vi "FrontPanel.vi"() -> ()   [LabVIEW 2013]
doc: "This VI controls the blindpanel type GHS-2T-1T-700 for a CryoFree DR. Automatization control is embedded in the blindpanel. Keys can be manipulated from within this VI."
uses:
  Lib/Lib.llb/ErrCodeStatusLkup.vi
  Lib/Lib.llb/Pfeiffer Vacuum.lvlib
panel:
  out "millisecond timer value":u32
  out "Timer 2":u32
  out "Timer 1":u32
  out "Cur Path":path
  in  "Start":bool caption="stop"
  in  "stop":bool
  in  "Side Panel":enum32{"Main", "HW Settings"}(tab)=enum."HW Settings"
  out "Sensors Status":T1={"String 8"="OK", "String 9"="OK", "String 10"="OK", "String 11"="OK", "String 12"="OK", "String 13"="OK"}
  out "cluster":T2 {"Channel 1" format="%-7.2e mbar"; "Channel 1" format="%-7.2e mbar"; "Channel 1" format="%-7.2e mbar"; "Channel 1" format="%-7.2e mbar"; "Channel 1" format="%-7.2e mbar"; "Channel 1" format="%-7.2e mbar"}
  out "Cluster":T3={"String 2"="\"\"", "String 3"="", "String 4"="", "String 5"="", "String 6"="", "String 7"=""}
  in  "S1":enum32{"Page 1"}(tab)
  out "Error code":string
  in  "Reset Error":bool
  out "Turbo T":T4
  out "Turbo IW":cluster{"I:":string, "P:":string}
  out "Turbo status":T5={"uA"="000", "Set Speed"=FALSE, "On"=FALSE, "Error"=FALSE}
  in  "S2":enum32{"Page 1"}(tab)
  out "Error code":string
  in  "Reset Error 2":bool
  out "Turbo T 2":T4
  out "Turbo IW 2":cluster{"I:":string, "P:":string}
  out "Turbo status 2":T5={"uA"="000", "Set Speed"=FALSE, "On"=FALSE, "Error"=FALSE}
  in  "Data Logging \nOptions":T6={"Plot data "=TRUE, "Every"=1.0, "Save to log"=TRUE, "Every  2"=1.0, "AVS_Path 2"=path "C:/avs-47", "AVS_FName"="logFP", "Filename suffix"="_%Y-%m-%d-%H-%M-%S", "NewFevery"=7, "Time Units"=enum."Days", "Date Format"="%Y-%m-%d %H:%M:%S", "Averages"=4} {"Every  2" format="%#_g min"; "Every" format="%#_g min"}
  in  "P6&7 Settings":T7={"P6 low"=20, "P6 high"=1600, "P7 low"=20, "P7 high"=1610, "Delay preset"=86400.0} {"Delay preset" format="%#_g minutes"}
  in  "P5 Settings":cluster{"P6 low":u16, "P6 high":u16}={"P6 low"=20, "P6 high"=1000}
  in  "NCP5 Settings":T8={"P6 low"=20, "P6 high"=1000, "P7 low"=20}
  out "P6&7 limits":T9={"P6 low"=20, "P6 high"=20, "P7 low"=20, "P7 high"=20}
  out "P5 limits":cluster{"P5 low":u16, "P5 high":u16}={"P5 low"=20, "P5 high"=20}
  out "NCP5 limits":T10={"P5 low"=20, "P5 med"=20, "P5 high"=20}
  in  "SET VALUES":bool
  in  "ADC Scaling":T11={"Front panel ADC scaling factors"={"P1"=2500.0, "P2"=2500.0, "P3"=2500.0, "P4"=2500.0, "P5"=2500.0, "P6"=2500.0, "P7"=2500.0, "Flow meter"=256.0, "PC"=10000.0}} {"Front panel ADC scaling factors"."Flow meter" format="%#.4f"}
  in  "Configuration":T12={"FP port"="COM7", "MG port"="COM9", "PT Enabled?"=FALSE, "MG  channel P8"=65535, "Stop auto recovery if still is empty"=FALSE, "PT port"="COM2", "MG Enabled?"=FALSE, "Type"=enum."Wet", "Slave Address"=16, "S1 Enabled?"=FALSE, "S1 port"="COM2", "S2 Enabled?"=FALSE, "S2 port"="COM2", "Device address S1"=1, "Device address S2"=2} {"MG  channel P8" items=["Channel 1", "Channel 2", "Channel 3", "Channel 4", "Channel 5", "Channel 6"]; "Slave Address" min=16 max=126 step=1}
  in  "Error Panel":enum32{"Page 1", "Page 2"}(tab)
  out "PT error":errorcluster
  out "FP error":errorcluster
  out "Sensor ERROR":string="No error"
  out "MaxiGauge ERROR":string="No error"
  out "MG error":errorcluster
  in  "Autoconf":bool caption="Autoconfigure"
  out "MG Data":dbl[](array[numeric]) format="%.3e"
  out "FP Data":sgl[](array[numeric]) format="%.2f"
  out "FP Status bits":u32[](array[numeric])
  out "Maxigauge ID":string
  out "PT Data":dbl[](array[numeric])
  in  "Pressures Panel":enum32{"Page 1", "Page 2"}(tab)
  out "PC":sgl format="%.1f"
  out "P1":sgl format="%.1f"
  out "P2":sgl format="%.1f"
  out "P3":sgl format="%.1f"
  out "P4":sgl format="%.1f"
  out "P5":sgl format="%.1f"
  out "P6":sgl format="%.1f"
  out "P7":sgl format="%.1f"
  out "Flow":sgl format="%#_4f"
  out "P5 Alarm":bool
  out "Pstill (P8)":dbl format="%.3f"
  out "Attempts Counter":u16
  in  "Main Panel":T13(tab)
  out "String":string
  out "String 3":string
  out "Mode":u16(ring) items=["AUTO MODE OFF", "START", "CONDENSING 3He", "CONDENSING 4He", "NORMAL CIRCULATION", "RECOVERY OF THE MIXTURE", "RECOVERY: BLOCKAGE OR OVERPRESSURE"]
  out "FLOW":sgl format="%#_3f"
  out "P5":sgl
  out "P4":sgl
  out "P3":sgl
  out "P1":sgl
  out "P2":sgl
  out "3He":sgl(slide) min=0 max=2 scale=0.0..2000.0 scale format="%.2f"
  out "4He":sgl(slide) min=0 max=2 scale=0.0..2000.0 scale format="%.2f"
  out "Panel ID":string
  out "Revision":string caption="V"
  in  "Tab Control 4":enum32{"OLD", "NEW"}(tab)
  in  "Buttons":T14
  out "LEDs":T15
  out "PC":sgl caption="P COMP"
  in  "Buttons 2":T14
  out "LEDs 2":T16
  in  "PT Plots Select":T17
  out "PT Error Code":i32
  out "PT Status":string="NO ERROR"
  in  "Time delay":u16=60 format="%.0f s"
  in  "Attempts":u16=6
  in  "Restart PT on Error?":bool
  in  "Reset MIN/MAX":bool
  out "Motor Current":i32(slide) scale=0.0..50.0 scale format="%#.0f"
  out "He Pressure":cluster{dbl, dbl, dbl, dbl, dbl, dbl}(knob) scale=0.0..400.0
  out "Oil Temp":cluster{dbl, dbl, dbl, dbl}(slide)={0.0, 0.0, 0.0, 48.8} scale=0.0..55.0
  out "He Temp":cluster{dbl, dbl, dbl, dbl}(slide)={0.0, 0.0, 0.0, 87.8} scale=0.0..95.0
  out "Out Water Temp":cluster{dbl, dbl, dbl, dbl}(slide)={0.0, 0.0, 0.0, 52.0} scale=0.0..60.0
  in  "PT start":bool
  in  "PT stop":bool
  out "In Water Temp":cluster{dbl, dbl, dbl, dbl}(slide)={0.0, 0.0, 0.0, 29.4} scale=0.0..35.0
  out "PT Control":u16(ring) items=["Compressor OFF", "Compressor ON", ""]
  out "Error Log":string[][](table)
  out "PT Status":cluster{"Time":dbl[], "Value":dbl[]}[](graph)
  in  "MG Plots Select":T17
  in  "FP Plots Select":T17
  out "MaxiGauge":cluster{"Time":dbl[], "Value":dbl[]}[](graph)
  out "Front Panel":cluster{"Time":dbl[], "Value":dbl[]}[](graph)
  # "MaxiGauge"
  # "#"
  # "Name"
  # "Pressure"
  # "Status"
  # "1"
  # "2"
  # "3"
  # "4"
  # "5"
  # "6"
  # "Turbo1 (S1)"
  # "°C"
  # "°C"
  # "°C"
  # "°C"
  # "°C"
  # "A"
  # "W"
  # "Hz"
  # "Turbo2 (S2)"
  # "°C"
  # "°C"
  # "°C"
  # "°C"
  # "°C"
  # "A"
  # "W"
  # "Hz"
  # "Data Logging and Plotting"
  # "Automatic mode pressure limits"
  # "Warning: these values influence the automatic \nmode operation of the GHS. Please consult with Leiden Cryogenics before changing them."
  # "Front panel ADC scaling factors"
  # "NAME"
  # "EPROM"
  # "NEW"
  # "DESCRIPTION"
  # "Stop condensing 4He"
  # "Stop recovering 4He"
  # "Stop condensing 3He"
  # "Stop recovering 3He"
  # "Condensing->open 12"
  # "Condensing->close 9/12"
  # "NC->open second line"
  # "NC->start MC"
  # "NC->open aux. trap"
  # "MaxiGauge"
  # "Pulse Tube"
  # "Turbo 1 (S1) (Pfeiffer HiPACE only)"
  # "Turbo2 (S2) (Pfeiffer HiPACE only)"
  # "Front Panel"
  # "Front Panel Status"
  # "MaxiGauge Status"
  # "Pulse Tube Status"
  # "Leiden Cryogenics"
  # "to 3He\nin-1"
  # "to 3He\nin-2"
  # "from still"
  # "to \nair"
  # "N.C."
  # "from\novc"
  # "from\nivc"
  # "P8"
  # "AUX 1"
  # "MIXTURE\nCOMPRESSOR"
  # "M2"
  # "P6"
  # "M3"
  # "M1"
  # "AUX PORT-1"
  # "P7"
  # "TRAP"
  # "AUX TRAP"
  # "to 3He\nin-1"
  # "to 3He\nin-2"
  # "from still"
  # "To \nAir"
  # "From\nIVC"
  # "to 3He\nin-1"
  # "to 3He\nin-2"
  # "from still"
  # "to \nair"
  # "N.C."
  # "from\novc"
  # "from\nivc"
  # "Leiden Cryogenics"
  # "to 3He\nin-1"
  # "to 3He\nin-2"
  # "from still"
  # "to \nair"
  # "N.C."
  # "from\novc"
  # "from\nivc"
  # "P8"
  # "P8"
  # "M2"
  # "P6"
  # "M3"
  # "TRAP"
  # "AUX TRAP"
  # "M1"
  # "AUX PORT-1"
  # "P7"
  # "to 3He\nin-1"
  # "to 3He\nin-2"
  # "from still"
  # "To \nAir"
  # "From\nIVC"
  # "to 3He\nin-1"
  # "to 3He\nin-2"
  # "from still"
  # "to \nair"
  # "N.C."
  # "from\novc"
  # "from\nivc"
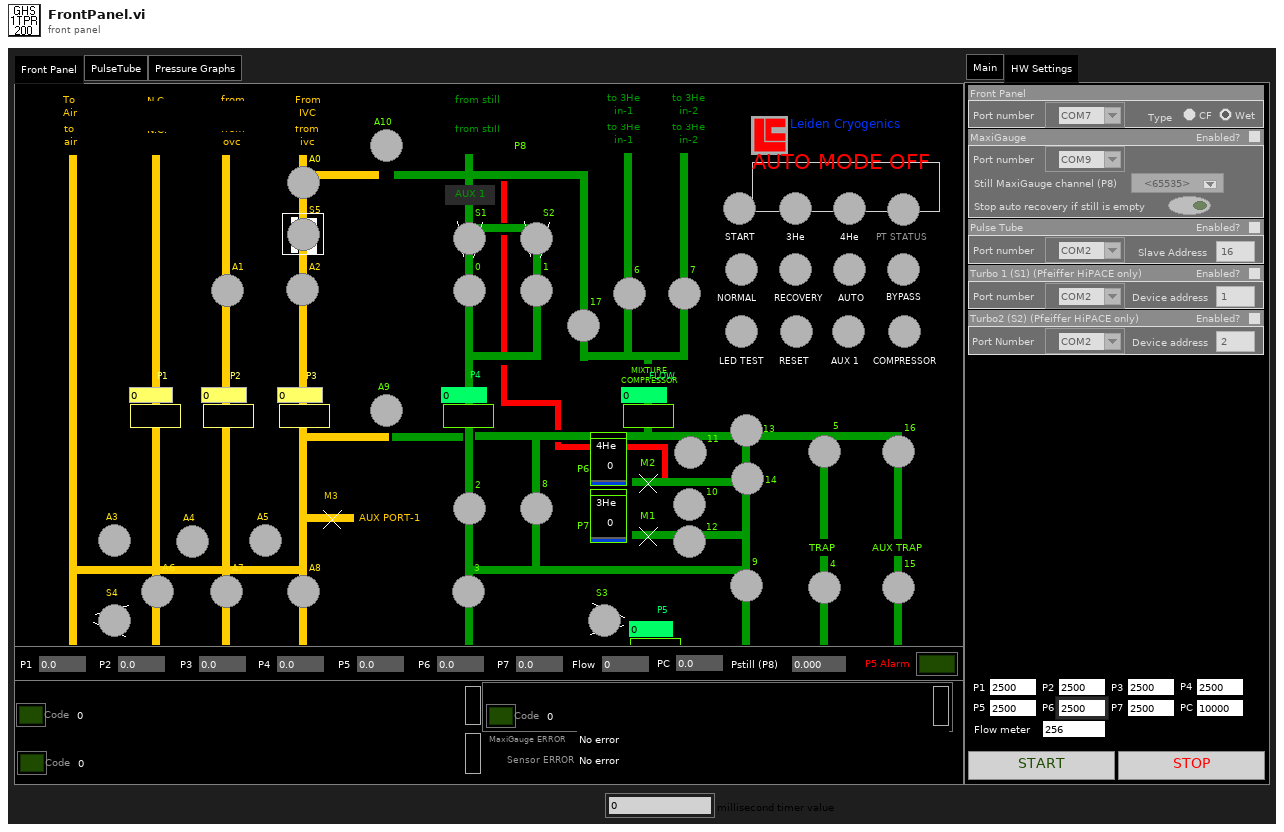
[diagram p1: front panel]
types:
  T1 = cluster{"String 8":string, "String 9":string, "String 10":string, "String 11":string, "String 12":string, "String 13":string}
  T2 = cluster{"Channel 1":dbl, "Channel 1":dbl, "Channel 1":dbl, "Channel 1":dbl, "Channel 1":dbl, "Channel 1":dbl}
  T3 = cluster{"String 2":string, "String 3":string, "String 4":string, "String 5":string, "String 6":string, "String 7":string}
  T4 = cluster{"Inverter":string, "Electronics":string, "Pump":string, "Bearing":string, "Motor":string}
  T5 = cluster{"uA":string, "Set Speed":bool, "On":bool, "Error":bool}
  T6 = cluster{"Plot data ":bool, "Every":dbl, "Save to log":bool, "Every  2":dbl, "AVS_Path 2":path, "AVS_FName":string, "Filename suffix":string, "NewFevery":u32, "Time Units":enum16{"Minutes", "Hours", "Days"}, "Date Format":string, "Averages":i32}
  T7 = cluster{"P6 low":u16, "P6 high":u16, "P7 low":u16, "P7 high":u16, "Delay preset":dbl}
  T8 = cluster{"P6 low":u16, "P6 high":u16, "P7 low":u16}
  T9 = cluster{"P6 low":u16, "P6 high":u16, "P7 low":u16, "P7 high":u16}
  T10 = cluster{"P5 low":u16, "P5 med":u16, "P5 high":u16}
  T11 = cluster{"Front panel ADC scaling factors":cluster{"P1":dbl, "P2":dbl, "P3":dbl, "P4":dbl, "P5":dbl, "P6":dbl, "P7":dbl, "Flow meter":dbl, "PC":dbl}}
  T12 = cluster{"FP port":refnum<visa-resource-name>, "MG port":refnum<visa-resource-name>, "PT Enabled?":bool, "MG  channel P8":u16, "Stop auto recovery if still is empty":bool, "PT port":refnum<visa-resource-name>, "MG Enabled?":bool, "Type":enum32{"CF", "Wet"}, "Slave Address":u8, "S1 Enabled?":bool, "S1 port":refnum<visa-resource-name>, "S2 Enabled?":bool, "S2 port":refnum<visa-resource-name>, "Device address S1":u8, "Device address S2":u8}
  T13 = enum32{"Front Panel", "PulseTube", "Pressure Graphs"}
  T14 = cluster{"baux2":bool, "bBypass":bool, "b15":bool, "b16":bool, "NC 0":bool, "baux1":bool, "b4":bool, "NC 1":bool, "b5":bool, "breset":bool, "NC 2":bool, "b9":bool, "b14":bool, "NC 3":bool, "b13":bool, "bledtest":bool, "NC 4":bool, "b12":bool, "b10":bool, "NC 5":bool, "b11":bool, "bA0":bool, "NC 9":bool, "b7":bool, "bS3":bool, "NC 12":bool, "b6":bool, "b17":bool, "NC 13":bool, "b8":bool, "b1":bool, "NC 14":bool, "bS2":bool, "b3":bool, "NC 15":bool, "b2":bool, "b0":bool, "NC 16":bool, "bS1":bool, "bA9":bool, "NC 17":bool, "bA8":bool, "bA2":bool, "NC 6":bool, "bs5":bool, "bA10":bool, "NC 7":bool, "bstart":bool, "bA5":bool, "NC 8":bool, "bA7":bool, "bA1":bool, "NC 10":bool, "bauto":bool, "bA4":bool, "NC 11":bool, "bA6":bool, "bS4":bool, "NC 18":bool, "bA3":bool, "b3he":bool, "b4he":bool, "bnorm":bool, "brecov":bool}
  T15 = cluster{"COMPR/AUX 2":bool, "BYPASS":bool, "15":bool, "16":bool, "NC 0":bool, "AUX 1":bool, "4":bool, "NC 1":bool, "5":bool, "RESET":bool, "NC 2":bool, "9":bool, "14":bool, "NC 3":bool, "13":bool, "LED TEST":bool, "NC 4":bool, "12":bool, "10":bool, "NC 5":bool, "11":bool, "A0":bool, "NC 12":bool, "7":bool, "S3":bool, "NC 13":bool, "6":bool, "17":bool, "NC 14":bool, "8":bool, "1":bool, "NC 15":bool, "S2":bool, "3":bool, "NC 16":bool, "2":bool, "0":bool, "NC 17":bool, "S1":bool, "A9":bool, "NC 6":bool, "A8":bool, "A2":bool, "NC 7":bool, "S5":bool, "A10":bool, "NC 8":bool, "START":bool, "A5":bool, "NC 9":bool, "A7":bool, "A1":bool, "NC 10":bool, "AUTO":bool, "A4":bool, "NC 11":bool, "A6":bool, "S4":bool, "NC 18":bool, "A3":bool, "3He":bool, "4He":bool, "NORMAL":bool, "RECOVERY":bool, "PT STATUS":bool}
  T16 = cluster{"COMPR/AUX 2":bool, "BYPASS":bool, "15":bool, "16":bool, "NC 0":bool, "GATE\nVALVE":bool, "4":bool, "NC 1":bool, "5":bool, "RESET":bool, "NC 2":bool, "9":bool, "14":bool, "NC 3":bool, "13":bool, "LED TEST":bool, "NC 4":bool, "12":bool, "10":bool, "NC 5":bool, "11":bool, "A0":bool, "NC 12":bool, "7":bool, "S3":bool, "NC 13":bool, "6":bool, "17":bool, "NC 14":bool, "8":bool, "1":bool, "NC 15":bool, "S2":bool, "3":bool, "NC 16":bool, "2":bool, "0":bool, "NC 17":bool, "S1":bool, "A9":bool, "NC 6":bool, "A8":bool, "A2":bool, "NC 7":bool, "S5":bool, "A10":bool, "NC 8":bool, "START":bool, "A5":bool, "NC 9":bool, "A7":bool, "A1":bool, "NC 10":bool, "AUTO":bool, "A4":bool, "NC 11":bool, "A6":bool, "S4":bool, "NC 18":bool, "A3":bool, "3He":bool, "4He":bool, "NORMAL":bool, "RECOVERY":bool, "PT STATUS":bool}
  T17 = cluster{"Boolean":bool, "Boolean 2":bool, "Boolean 3":bool, "Boolean 4":bool, "Boolean 5":bool, "Boolean 6":bool, "Boolean 7":bool, "Boolean 8":bool}
  T18 = cluster{"error":bool, "code":i32, "source":string}
  T19 = cluster{"type":string, "creator":string, "permissions":i32, "data size":i32, "res size":i32, "creation date":u32, "modification date":u32, "bFolder":bool, "bInvisible":bool, "location":cluster{"vertical":i16, "horizontal":i16}, "owner":string, "group":string}
  T20 = cluster{"FP Data[0]":sgl, "FP Data[1]":sgl, "FP Data[2]":sgl, "FP Data[3]":sgl, "FP Data[4]":sgl, "FP Data[5]":sgl, "FP Data[6]":sgl, "FP Data[7]":sgl, "FP Data[8]":sgl}
  T21 = enum32{"invalid app kind", "Development System", "Run Time System", "Student Edition", "Embedded LabVIEW", "Evaluation", "Custom"}
  T22 = enum32{"HKEY_CLASSES_ROOT", "HKEY_CURRENT_USER", "HKEY_LOCAL_MACHINE", "HKEY_USERS", "HKEY_PERFORMANCE_DATA", "HKEY_CURRENT_CONFIG", "HKEY_DYN_DATA"}
  T23 = cluster{"Array[0]":string, "Array[1]":string, "Array[2]":string, "Array[3]":string, "Array[4]":string, "Array[5]":string}
  T24 = cluster{"array of 4 x 16 bit unsigned[0]":u16, "array of 4 x 16 bit unsigned[1]":u16, "array of 4 x 16 bit unsigned[2]":u16, "array of 4 x 16 bit unsigned[3]":u16}
  T25 = cluster{"[0]":u32, "[1]":u32, "[2]":u32, "[3]":u32, "[4]":u32}
  T26 = cluster{"array of 2 x 16 bit unsigned[0]":u16, "array of 2 x 16 bit unsigned[1]":u16}
  T27 = cluster{"array of 3 x 16 bit unsigned[0]":u16, "array of 3 x 16 bit unsigned[1]":u16, "array of 3 x 16 bit unsigned[2]":u16}
  T28 = cluster{"[0]":bool, "[1]":bool, "[2]":bool, "[3]":bool, "[4]":bool, "[5]":bool, "[6]":bool, "[7]":bool, "[8]":bool, "[9]":bool, "[10]":bool, "[11]":bool, "[12]":bool, "[13]":bool, "[14]":bool, "[15]":bool, "[16]":bool, "[17]":bool, "[18]":bool, "[19]":bool, "[20]":bool, "[21]":bool, "[22]":bool, "[23]":bool, "[24]":bool, "[25]":bool, "[26]":bool, "[27]":bool, "[28]":bool, "[29]":bool, "[30]":bool, "[31]":bool, "[32]":bool, "[33]":bool, "[34]":bool, "[35]":bool, "[36]":bool, "[37]":bool, "[38]":bool, "[39]":bool, "[40]":bool, "[41]":bool, "[42]":bool, "[43]":bool, "[44]":bool, "[45]":bool, "[46]":bool, "[47]":bool, "[48]":bool, "[49]":bool, "[50]":bool, "[51]":bool, "[52]":bool, "[53]":bool, "[54]":bool, "[55]":bool, "[56]":bool, "[57]":bool, "[58]":bool, "[59]":bool, "[60]":bool, "[61]":bool, "[62]":bool, "[63]":bool, "[64]":bool}
  T29 = cluster{"P1":dbl, "P2":dbl, "P3":dbl, "P4":dbl, "P5":dbl, "P6":dbl, "P7":dbl, "Flow meter":dbl, "PC":dbl}
  T30 = cluster{"Dict. Var":u16, "Description":string, "Values":i32[]}[]
  T31 = cluster{"[3]":dbl, "[3]":dbl, "[3]":dbl, "Values[3] 2":dbl}
  T32 = cluster{"[0]":dbl, "[0]":dbl, "[0]":dbl, "[1]":dbl, "[1]":dbl, "[1]":dbl}
  T33 = cluster{"[2]":dbl, "[2]":dbl, "[2]":dbl, "Values[2] 2":dbl}
  T34 = cluster{"[1]":dbl, "[1]":dbl, "[1]":dbl, "Values[1] 2":dbl}
  T35 = cluster{"Values[0]":dbl, "Values[0]":dbl, "Values[0]":dbl, "Values[0] 2":dbl}
  T36 = cluster{"Speed":string, "Set Speed":bool, "On":bool, "Error":bool}
  T37 = cluster{"error":bool, "code":i32, "error source":string}
  T38 = cluster{"sensor status info[0]":string, "sensor status info[1]":string, "sensor status info[2]":string, "sensor status info[3]":string, "sensor status info[4]":string, "sensor status info[5]":string}
  T39 = cluster{"Filterred[0]":dbl, "Filterred[1]":dbl, "Filterred[2]":dbl, "Filterred[3]":dbl, "Filterred[4]":dbl, "Filterred[5]":dbl}
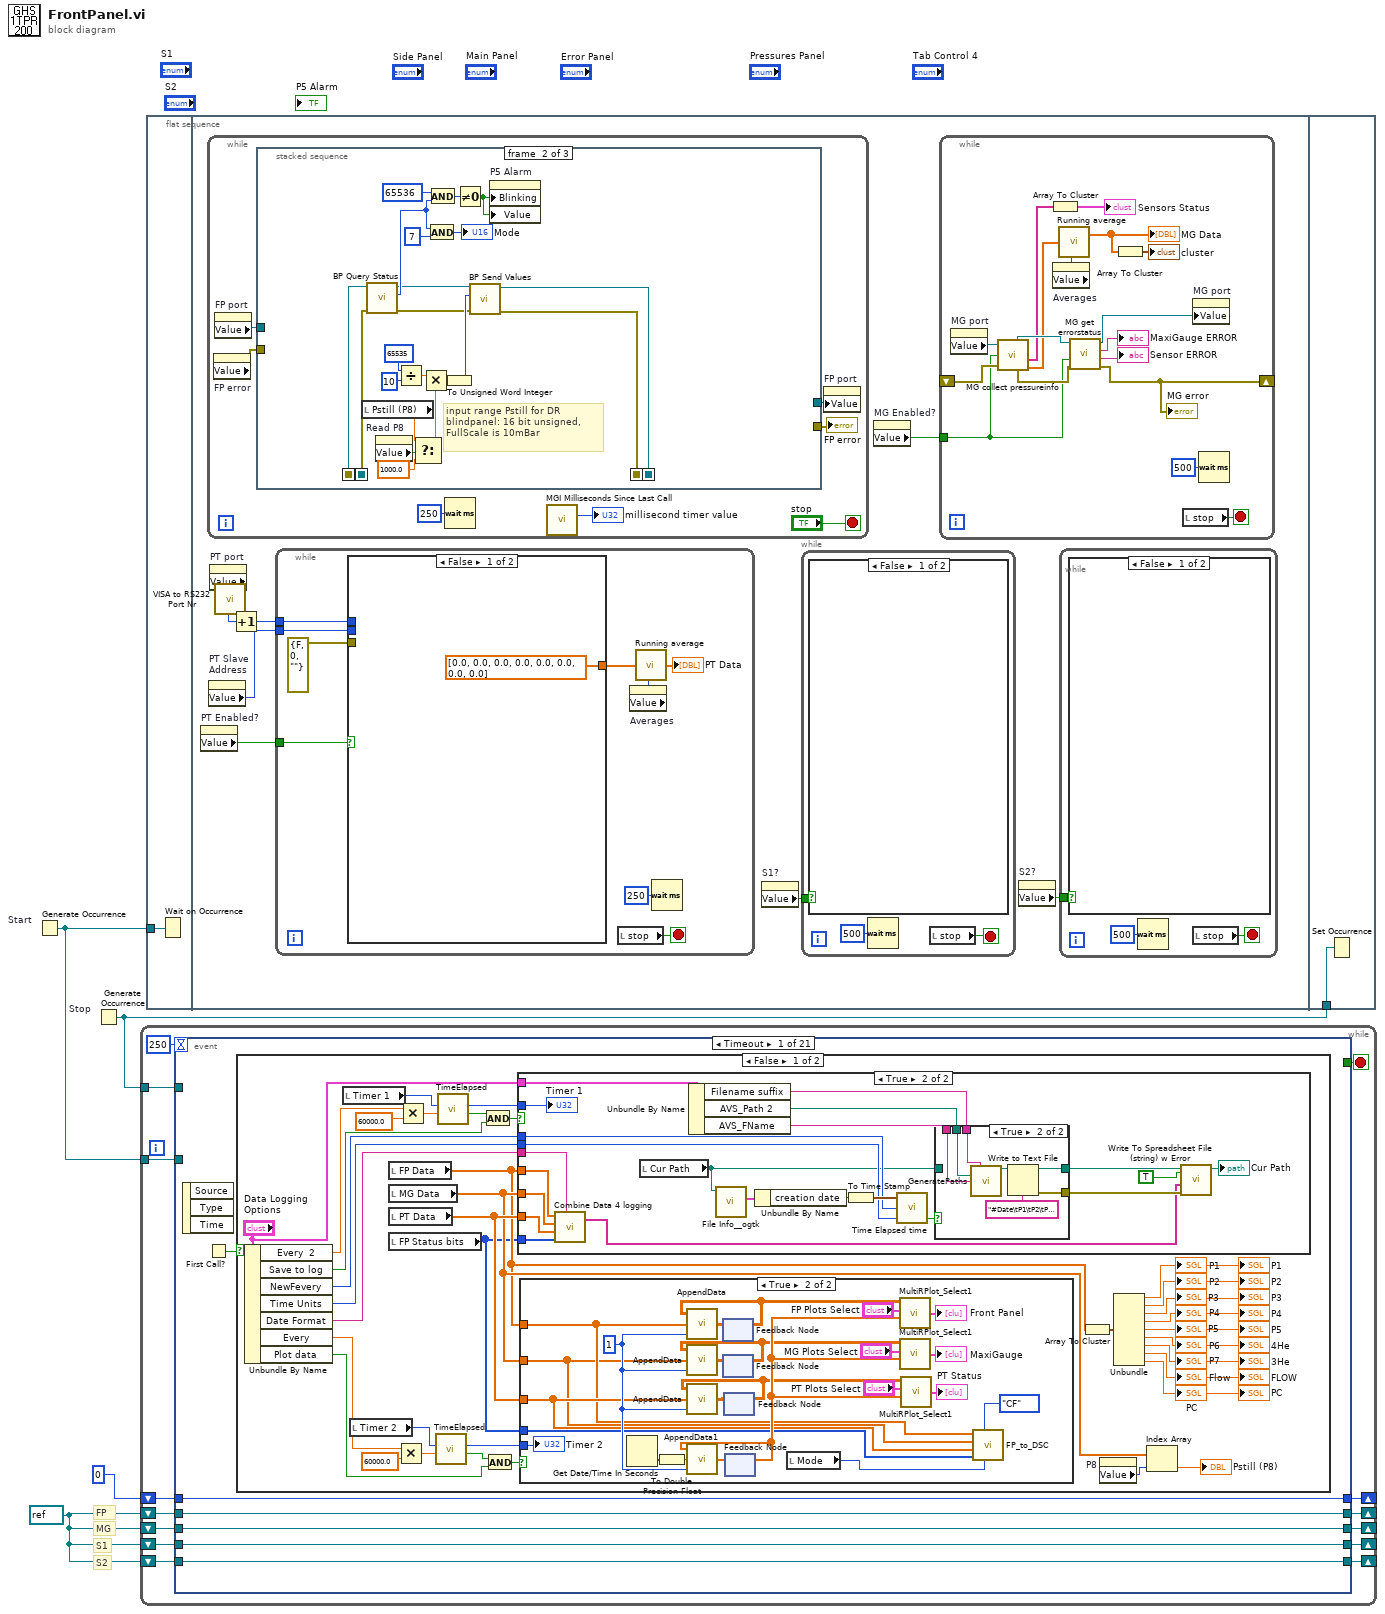
[diagram p0: block diagram]
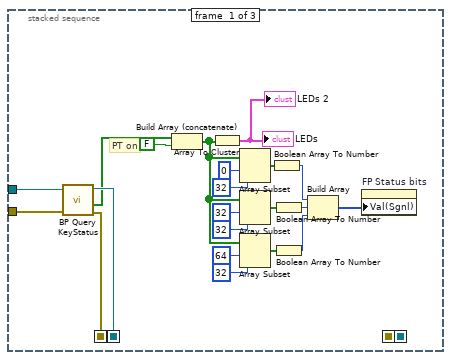
[diagram p2: hidden frame]
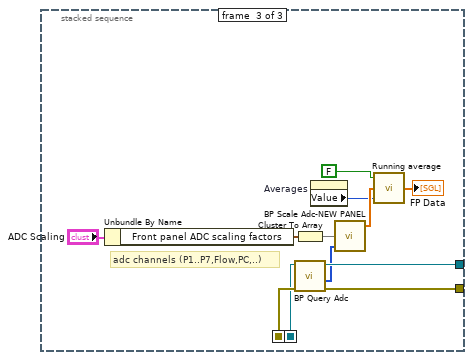
[diagram p3: hidden frame]
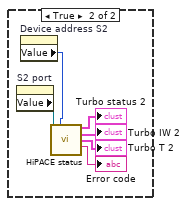
[diagram p4: hidden frame]
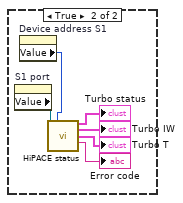
[diagram p5: hidden frame]
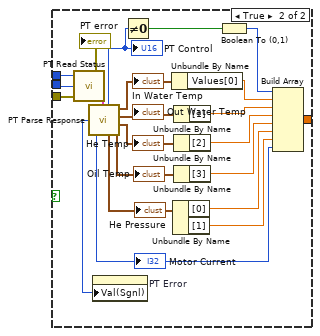
[diagram p6: hidden frame]
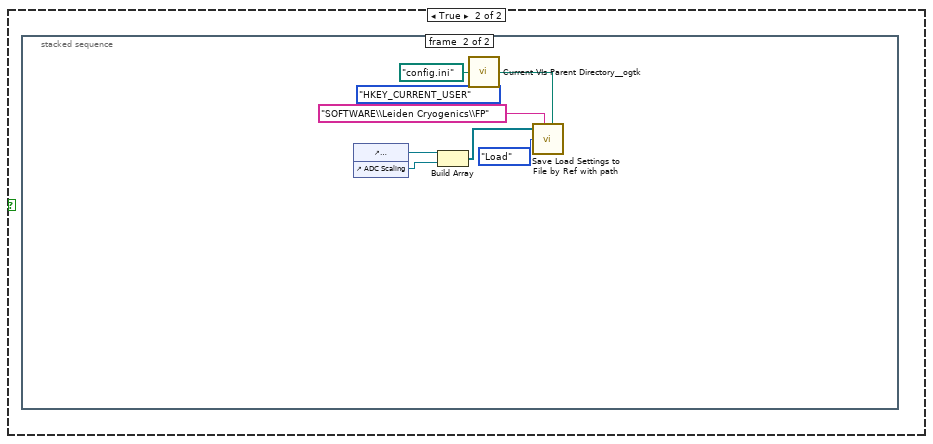
[diagram p10: hidden frame]
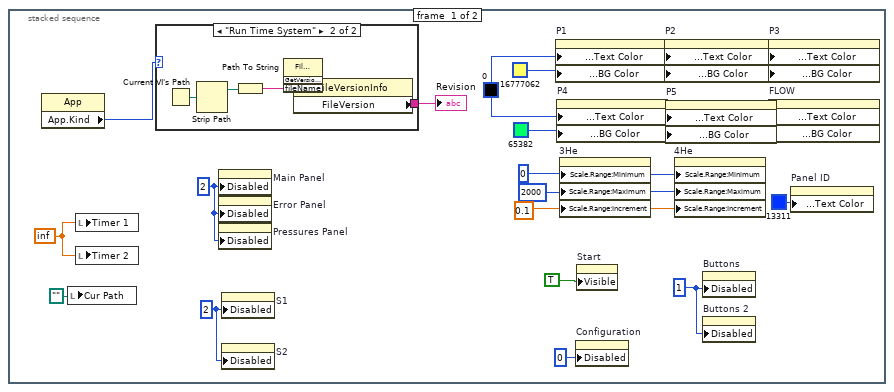
[diagram p11: hidden frame]
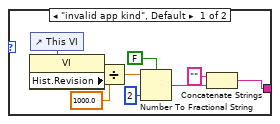
[diagram p12: hidden frame]
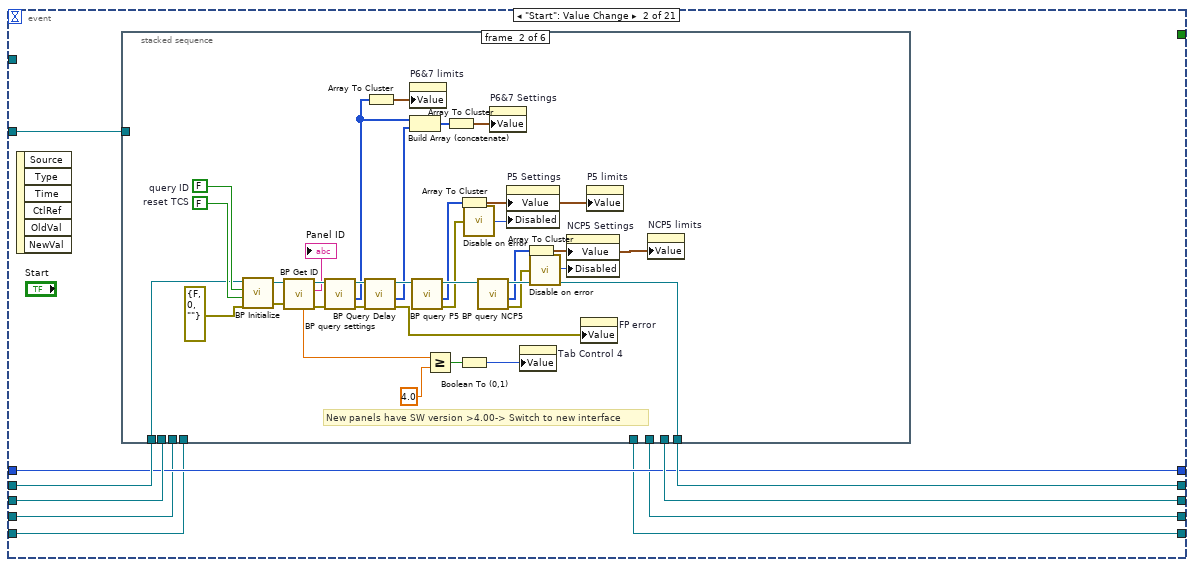
[diagram p13: hidden frame]
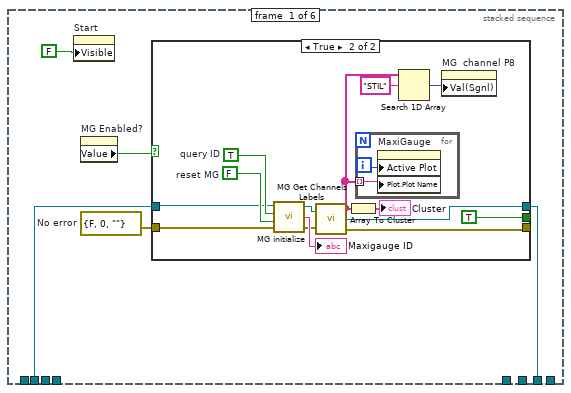
[diagram p14: hidden frame]
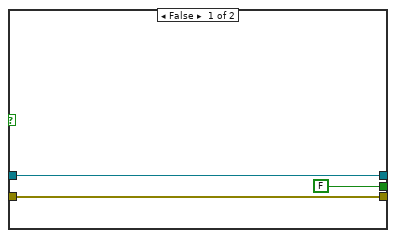
[diagram p15: hidden frame]
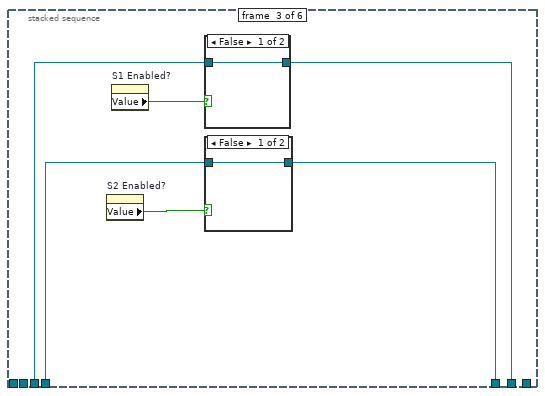
[diagram p16: hidden frame]
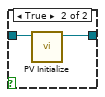
[diagram p17: hidden frame]
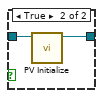
[diagram p18: hidden frame]
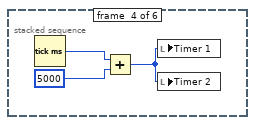
[diagram p19: hidden frame]
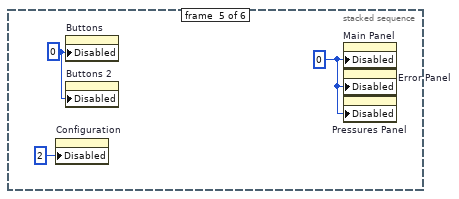
[diagram p20: hidden frame]
diagram:
  w2 = refnum<visa-resource-name> refnum ("PT port")
  # "S2"
  # "S1"
  # "FP"
  # "MG"
  n1 = Generate Occurrence "Start"() -> (w4:refnum<k4>)
  n2 = Generate Occurrence "Stop"() -> (w1:refnum<k4>)
  n3 = while {
    shift-right: [w10] -> _
    shift-left: w2 -> [w16]
    shift-right: [w14] -> _
    shift-left: w2 -> [w15]
    tunnel: w4 -> [w13]
    shift-right: [w11] -> _
    shift-left: 0 -> [w12]
    shift-right: [w7] -> _
    shift-left: w2 -> [w9]
    shift-right: [w6] -> _
    shift-left: w2 -> [w8]
    tunnel: w1 -> [w5]
    stop <- w18 stop-if-true
    n4 = event shown="[0] Timeout" {
      selector: _ -> [_ _ _ _ _ _ _ _ _ _ _ _ _ _ _ _ _ _ _ _ _]
      dyn-events: _ -> [_ _ _ _ _ _ _ _ _ _ _ _ _ _ _ _ _ _ _ _ _]
      timeout: 250 -> [_ _ _ _ _ _ _ _ _ _ _ _ _ _ _ _ _ _ _ _ _]
      tunnel: [_ _ TRUE _ _ _ _ _ _ _ _ _ _ _ _ _ _ _ _ _ _] -> w18
      tunnel: w16 -> [w23 w158 w240 w261 w268 w280 w291 w302 w330 w355 w363 w371 w387 w405 w410 w420 w427 w466 w472 w479 w489]
      tunnel: w15 -> [w21 w160 w239 w260 w266 w278 w290 w301 w329 w354 w362 w370 w388 w404 w409 w419 w426 w467 w473 w478 w488]
      tunnel: [w21 w159 _ w260 w266 w278 w290 w301 w329 w354 w362 w370 w377 w404 w409 w419 w426 w467 w473 w478 w488] -> w14
      tunnel: w13 -> [_ w156 _ _ _ _ _ _ _ _ _ _ _ _ _ _ _ _ _ _ _]
      tunnel: w12 -> [w22 w155 _ w259 w265 w277 w289 w298 w328 w353 w361 w372 _ w406 w411 w418 w428 w465 w471 w480 w490]
      tunnel: [w22 w155 _ w259 w265 w277 w289 w298 w328 w353 w361 w372 w389 w406 w411 w418 w428 w465 w471 w480 w490] -> w11
      tunnel: [w23 w157 _ w261 w267 w279 w291 w302 w330 w338 w363 w371 w392 w405 w410 w420 w427 w466 w472 w479 w489] -> w10
      tunnel: w9 -> [w20 w154 w238 w258 w264 w276 w288 w294 w327 w352 w360 w369 w376 w403 w408 w417 w425 w469 w474 w477 w487]
      tunnel: w8 -> [w19 w153 w237 w257 w263 w275 w287 w293 w326 w351 w359 w368 w374 w402 w407 w416 w424 w468 w475 w476 w486]
      tunnel: [w20 w152 _ w258 w264 w276 w288 w294 w327 w352 w360 w369 w375 w403 w408 w417 w425 _ w474 w477 w487] -> w7
      tunnel: [w19 w151 _ w257 w263 w275 w287 w293 w326 w351 w359 w368 w373 w402 w407 w416 w424 w468 _ w476 w486] -> w6
      tunnel: w5 -> [_ _ w236 _ _ _ _ _ _ _ _ _ _ _ _ _ _ _ _ _ _]
      event Timeout {
        n5 = event-data() -> ()  [unwired: 1 in, 3 out]
        n6 = First Call?() -> (First Call?: T/F=w24:bool)
        n7 = case shown="False" w24 {
          frame False {
            n8 = Unbundle By Name("Data Logging \nOptions") -> ("Every  2"=w41:dbl, "Save to log"=w42:bool, "NewFevery"=w40:u32, "Time Units"=w39:enum16{"Minutes", "Hours", "Days"}, "Date Format"=w35:string, "Every"=w43:dbl, "Plot data"=w44:bool)
            n9 = local read "Timer 1"() -> (w29:u32)
            n10 = local read "Timer 2"() -> (w27:u32)
            n11 = local read "FP Data"() -> (w37:sgl[])
            n12 = local read "MG Data"() -> (w54:dbl[])
            n13 = local read "PT Data"() -> (w56:dbl[])
            n14 = local read "FP Status bits"() -> (w25:u32[])
            n15 = Multiply(x=w43, y=60000.0 ("Numeric")) -> (x*y=w32:dbl)
            n16 = Multiply(x=w41, y=60000.0) -> (x*y=w34:dbl)
            n17 = call "TimeElapsed.vi"("Numeric"=w32, "timer"=w27) -> ("Boolean"=w31:bool, "millisecond timer value"=w28:u32)  [unwired: 4 in]
            n18 = call "TimeElapsed.vi"("Numeric"=w34, "timer"=w29) -> ("Boolean"=w33:bool, "millisecond timer value"=w30:u32)  [unwired: 4 in]
            n19 = And(x=w33, y=w42) -> (x .and. y?=w60:bool)
            n20 = And(x=w31, y=w44) -> (x .and. y?=w57:bool)
            n21 = case shown="True" w60 {
              tunnel: w37 -> [_ w104]
              tunnel: w54 -> [_ w103]
              tunnel: w25 -> [_ w102]
              tunnel: w56 -> [_ w105]
              tunnel: w40 -> [_ w98]
              tunnel: w39 -> [_ w97]
              tunnel: "Data Logging \nOptions" -> [_ w93]
              tunnel: w35 -> [_ w87]
              tunnel: w30 -> [_ w85]
              frame False {
              }
              frame True {
                n22 = call "Combine Data 4 logging.vi"("FP Data"=w104, "MG Data"=w103, "PT Data"=w105, "FP Status Bits"=w102, "Time Format String"=w87) -> ("Array"=w89:string[])  [unwired: 1 in]
                n23 = local read "Cur Path"() -> (w86:path)
                n24 = Unbundle By Name(w93) -> ("Filename suffix"=w90:string, "AVS_Path 2"=w92:path, "AVS_FName"=w91:string)
                n25 = call "File Info__ogtk.vi"("file"=w86) -> ("file info"=w101:T19)  [unwired: 5 in, 2 out]
                n26 = Unbundle By Name(w101) -> ("creation date"=w100:u32)
                n27 = To Time Stamp(1:w100) -> (0:w99:timestamp)
                n28 = call "Time Elapsed time.vi"("Time Units"=w97, "Delay Time"=w98, "Time Old In"=w99) -> ("T>dT?"=w88:bool)  [unwired: 2 out]
                n29 = case shown="True" w88 {
                  tunnel: [w107 w108] -> w95
                  tunnel: [_ w113] -> w94
                  tunnel: w92 -> [_ w112]
                  tunnel: w91 -> [_ w111]
                  tunnel: w90 -> [_ w110]
                  tunnel: w86 -> [w107 _]
                  frame False {
                  }
                  frame True {
                    n30 = call "GeneratePaths.vi"("Filename Suffix"=w110, "AVS_Path"=w112, "AVS_FName"=w111) -> ("Generated Log path"=w108:path)  [unwired: 11 in, 1 out]
                    n31 = Write to Text File(file (use dialog)=w108, text="#Date\tP1\tP2\tP3\tP4\tP5\tP6\tP7\tFlow\tMG0\tMG1\tMG2\tMG3\tMG4\tMG5\tPT on\tW_in\tW_out\tHe\tOil\tP_low\tP_high\tPT current\tState0\tState1\tState2\r\n") -> (error out=w113:errorcluster)  [unwired: 2 in, 2 out]
                  }
                }
                n32 = call "Write To Spreadsheet File (string) w Error.vi"("append to file? (new file:F)"=TRUE, "error in"=w94, "1D data"=w89, "file path (dialog if empty)"=w95) -> ("new file path (Not A Path if cancelled)"=→"Cur Path":path)  [unwired: 6 in, 1 out]
                "Timer 1" <- w85
              }
            }
            n33 = case shown="True" w57 {
              tunnel: w54 -> [_ w64]
              tunnel: w37 -> [_ w65]
              tunnel: w56 -> [_ w66]
              tunnel: w28 -> [_ w67]
              tunnel: w25 -> [_ w62]
              frame False {
              }
              frame True {
                w68 = 1 ("Smoothing window")
                n34 = Get Date/Time In Seconds() -> (seconds since 1Jan1904=w82:timestamp)
                n35 = To Double Precision Float(number=w82) -> (double precision float=w81:dbl)
                n36 = feedback #1() -> (w71:sgl[][])  [unwired: 1 in]
                n37 = call "AppendData.vi"("Smoothing window"=w68, "Current Measurement"=w65, "Data In"=w71) -> ("Data Out"=w83:sgl[][])
                n38 = feedback-in #1(w83) -> ()
                n39 = feedback #2() -> (w70:sgl[][])  [unwired: 1 in]
                n40 = call "AppendData.vi"("Smoothing window"=w68, "Current Measurement"=w64, "Data In"=w70) -> ("Data Out"=w84:sgl[][])
                n41 = feedback-in #2(w84) -> ()
                n42 = feedback #3() -> (w69:sgl[][])  [unwired: 1 in]
                n43 = call "AppendData.vi"("Smoothing window"=w68, "Current Measurement"=w66, "Data In"=w69) -> ("Data Out"=w72:sgl[][])
                n44 = feedback-in #3(w72) -> ()
                n45 = feedback #4() -> (w73:dbl[])  [unwired: 1 in]
                n46 = call "AppendData1.vi"("Smoothing window"=w68, "Current Measurement"=w81, "Data In"=w73) -> ("Data Out"=w80:dbl[])
                n47 = feedback-in #4(w80) -> ()
                n48 = local read "Mode"() -> (w61:u16)
                n49 = call "MultiRPlot_Select1.vi"("Time"=w73, "FP Plots Select"="FP Plots Select", "Data In"=w71) -> ("Out Array"=→"Front Panel":cluster{"Time":dbl[], "Value":dbl[]}[])  [unwired: 1 in]
                n50 = call "MultiRPlot_Select1.vi"("Time"=w73, "FP Plots Select"="MG Plots Select", "Data In"=w70) -> ("Out Array"=→"MaxiGauge":cluster{"Time":dbl[], "Value":dbl[]}[])  [unwired: 1 in]
                n51 = call "MultiRPlot_Select1.vi"("Time"=w73, "FP Plots Select"="PT Plots Select", "Data In"=w69) -> ("Out Array"=→"PT Status":cluster{"Time":dbl[], "Value":dbl[]}[])  [unwired: 1 in]
                n52 = call "FP_to_DSC.vi"("Mode"=w61, "Enum"=enum16{"CF", "MNK"}."CF", "FP Status Bits"=w62, "PT Data"=w66, "MG Data"=w64, "FP Data"=w65) -> ()  [unwired: 6 in]
                "Timer 2" <- w67
              }
            }
            n53 = Array To Cluster(array=w37) -> (cluster=w55:T20)
            n54 = property on="P8" class="Ring (strict)"() -> ("Value"=w52:u16)  [unwired: 2 in, 2 out]
            n55 = Unbundle(w55) -> ("FP Data[0]"=→"P1" →"P1":sgl, "FP Data[1]"=→"P2" →"P2":sgl, "FP Data[2]"=→"P3" →"P3":sgl, "FP Data[3]"=→"P4" →"P4":sgl, "FP Data[4]"=→"P5" →"P5":sgl, "FP Data[5]"=→"P6" →"4He":sgl, "FP Data[6]"=→"P7" →"3He":sgl, "FP Data[7]"=→"Flow" →"FLOW":sgl, "FP Data[8]"=→"PC" →"PC":sgl)
            n56 = Index Array(array=w54, index=w52) -> (element=→"Pstill (P8)":dbl)
          }
          frame True {
            n57 = stacked-sequence {
              frame #0 {
                w115 = u8 2 ("Disabled")
                w114 = u8 2 ("Disabled")
                w118 = inf
                w117 = u8 1 ("Disabled")
                w122 = u32 16777062
                w127 = u32 65382
                w126 = u32 0
                w125 = 0.1
                w124 = 2000
                w123 = 0
                n58 = property class="App"() -> ("App.Kind"=w128:T21)  [unwired: 2 in, 2 out]
                n59 = local write "Cur Path"(path "") -> ()
                n60 = local write "Timer 1"(w118) -> ()
                n61 = local write "Timer 2"(w118) -> ()
                n62 = case shown="\"Run Time System\"" w128 {
                  tunnel: [w130 w139] -> w129
                  frame "invalid app kind", Default {
                    n63 = control-ref of="This VI"() -> (w131:refnum<vi>)
                    n64 = property class="VI"(reference=w131) -> ("Hist.Revision"=w132:u32)  [unwired: 1 in, 2 out]
                    n65 = Divide(x=w132, y=1000.0 ("x")) -> (x/y=w136:dbl)
                    n66 = Number To Fractional String(use system decimal point (T)=FALSE, number=w136, precision (6)=i16 2) -> (F-format string=w137:string)  [unwired: 1 in]
                    n67 = Concatenate Strings("" ("string"), w137) -> (w130:string)
                  }
                  frame "Run Time System" {
                    n68 = Current VI's Path() -> (path=w142:path)
                    n69 = Strip Path(path=w142) -> (stripped path=w143:path)  [unwired: 1 out]
                    n70 = Path To String(path=w143) -> (string=w141:string)
                    n71 = invoke class="FileVersionInfo" method="GetVersionInfo"("fileName"=w141) -> ("GetVersionInfo"=w140:refnum<k24>)  [unwired: 3 in, 3 out]
                    n72 = property class="FileVersionInfo"(reference=w140) -> ("FileVersion"=w139:string)  [unwired: 1 in, 2 out]
                  }
                }
                "Revision" <- w129
                n73 = property on="Main Panel" class="TabCtl (strict)"("Disabled"=w114) -> ()  [unwired: 2 in, 2 out]
                n74 = property on="Error Panel" class="TabCtl (strict)"("Disabled"=w114) -> ()  [unwired: 2 in, 2 out]
                n75 = property on="Pressures Panel" class="TabCtl (strict)"("Disabled"=w114) -> ()  [unwired: 2 in, 2 out]
                n76 = property on="S1" class="TabCtl (strict)"("Disabled"=w115) -> ()  [unwired: 2 in, 2 out]
                n77 = property on="S2" class="TabCtl (strict)"("Disabled"=w115) -> ()  [unwired: 2 in, 2 out]
                n78 = property on="P1" class="DigNum (strict)"("Numeric Text.Text Colors:Text Color"=w126, "Numeric Text.Text Colors:BG Color"=w122) -> ()  [unwired: 2 in, 2 out]
                n79 = property on="P4" class="DigNum (strict)"("Numeric Text.Text Colors:Text Color"=w126, "Numeric Text.Text Colors:BG Color"=w127) -> ()  [unwired: 2 in, 2 out]
                n80 = property on="3He" class="Slide (strict)"("Scale.Range:Minimum"=w123, "Scale.Range:Maximum"=w124, "Scale.Range:Increment"=w125) -> ()  [unwired: 2 in, 2 out]
                n81 = property on="Configuration" class="Clust (strict)"("Disabled"=u8 0) -> ()  [unwired: 2 in, 2 out]
                n82 = property on="Start" class="Bool"("Visible"=TRUE) -> ()  [unwired: 2 in, 2 out]
                n83 = property on="P2" class="DigNum (strict)"("Numeric Text.Text Colors:Text Color"=w126, "Numeric Text.Text Colors:BG Color"=w122) -> ()  [unwired: 2 in, 2 out]
                n84 = property on="P5" class="DigNum (strict)"("Numeric Text.Text Colors:Text Color"=w126, "Numeric Text.Text Colors:BG Color"=w127) -> ()  [unwired: 2 in, 2 out]
                n85 = property on="4He" class="Slide (strict)"("Scale.Range:Minimum"=w123, "Scale.Range:Maximum"=w124, "Scale.Range:Increment"=w125) -> ()  [unwired: 2 in, 2 out]
                n86 = property on="Buttons" class="Clust"("Disabled"=w117) -> ()  [unwired: 2 in, 2 out]
                n87 = property on="Buttons 2" class="Clust"("Disabled"=w117) -> ()  [unwired: 2 in, 2 out]
                n88 = property on="P3" class="DigNum (strict)"("Numeric Text.Text Colors:Text Color"=w126, "Numeric Text.Text Colors:BG Color"=w122) -> ()  [unwired: 2 in, 2 out]
                n89 = property on="FLOW" class="DigNum (strict)"("Numeric Text.Text Colors:Text Color"=w126, "Numeric Text.Text Colors:BG Color"=w127) -> ()  [unwired: 2 in, 2 out]
                n90 = property on="Panel ID" class="Str"("Text.Text Colors:Text Color"=u32 13311) -> ()  [unwired: 2 in, 2 out]
              }
              frame #1 {
                (unwired) T22."HKEY_CURRENT_USER" ("root key (HKEY_LOCAL_MACHINE) 2")
                n91 = control-ref of="Configuration"() -> (w147:refnum<vi>)
                n92 = control-ref of="ADC Scaling"() -> (w144:refnum<vi>)
                n93 = Build Array(w147, w144) -> (w149:refnum<vi>[])
                n94 = call "Current VIs Parent Directory__ogtk.vi"("Relative path (.)"=path "config.ini") -> ("Parent Directory (+ Relative)"=w145:path)  [unwired: 4 in]
                n95 = call "Save Load Settings to File by Ref with path.vi"("Array of Cluster References"=w149, "subkey"="SOFTWARE\\Leiden Cryogenics\\FP" ("subkey 2"), "Action"=enum8{"Load", "Save"}."Load", "configuration file path"=w145) -> ()  [unwired: 5 in, 1 out]
              }
            }
          }
        }
      }
      event "Start": Value Change {
        n96 = event-data() -> ()  [unwired: 1 in, 6 out]
        n97 = stacked-sequence {
          tunnel: w160 -> [w163 _ _ _ _ _]
          tunnel: [w162 _ _ _ _ _] -> w159
          tunnel: w158 -> [_ w212 _ _ _ _]
          tunnel: [_ w202 _ _ _ _] -> w157
          tunnel: w156 -> [_ _ _ _ _ w235]
          tunnel: w154 -> [_ _ w222 _ _ _]
          tunnel: w153 -> [_ _ w221 _ _ _]
          tunnel: [_ _ w217 _ _ _] -> w152
          tunnel: [_ _ w220 _ _ _] -> w151
          frame #0 {
            w165 = T18 {"error"=FALSE, "code"=0, "source"=""}  # No error
            n98 = property on="Start" class="Bool"("Visible"=FALSE) -> ()  [unwired: 2 in, 2 out]
            n99 = property on="MG Enabled?" class="Bool (strict)"() -> ("Value"=w164:bool)  [unwired: 2 in, 2 out]
            n100 = case shown="True" w164 {
              tunnel: [w168 w178] -> _
              tunnel: [w166 w176] -> w162
              tunnel: w165 -> [w168 w181]
              tunnel: [FALSE TRUE] -> _
              tunnel: w163 -> [w166 w172]
              frame False {
                # "MaxiGauge not connected"
              }
              frame True {
                w174 = TRUE  # query ID
                w173 = FALSE  # reset MG
                n101 = call "MG initialize.vi"("error in (no error)"=w181, "MG query errorstatus"=w173, "ID query"=w174, "MaxiGauge port"=w172) -> ("error out"=w179:errorcluster, "program ID"=→"Maxigauge ID":string, "MaxiGauge port"=w177:refnum<visa-resource-name>)
                n102 = call "MG Get Channels Labels.vi"("MaxiGauge port"=w177, "error out 2"=w179) -> ("Array"=w171:string[], "MaxiGauge port"=w176:refnum<visa-resource-name>, "error out"=w178:errorcluster)
                n103 = Array To Cluster(array=w171) -> (cluster=→"Cluster":T23)
                n104 = for {
                  tunnel: w171 -> [w183] mode=indexing
                  i -> [w184]
                  n105 = property on="MaxiGauge" class="XYGraph (strict)"("Active Plot"=w184, "Plot.Plot Name"=w183) -> ()  [unwired: 2 in, 2 out]
                }
                n106 = Search 1D Array(1D array=w171, element="STIL") -> (index of element=w169:i32)  [unwired: 1 in]
                n107 = property on="MG  channel P8" class="Ring (strict)"("Val(Sgnl)"=w169) -> ()  [unwired: 2 in, 2 out]
              }
            }
          }
          frame #1 {
            w215 = FALSE  # reset TCS
            w216 = FALSE  # query ID
            # "New panels have SW version >4.00-> Switch to new interface"
            n108 = call "BP Initialize.vi"("error in (no error)"=T18 {"error"=FALSE, "code"=0, "source"=""} ("error in"), "reset"=w215, "ID query"=w216, "FrontPanel port"=w212) -> ("error out"=w211:errorcluster, "FrontPanel port"=w213:refnum<visa-resource-name>)  [unwired: 1 out]
            n109 = call "BP Get ID.vi"("error in (no error)"=w211, "FrontPanel port"=w213) -> ("error out"=w210:errorcluster, "Device ID string"=→"Panel ID":string, "FrontPanel port"=w209:refnum<visa-resource-name>, "SW Version"=w207:dbl)  [unwired: 5 in, 1 out]
            n110 = call "BP query settings.vi"("error in"=w210, "FrontPanel port"=w209) -> ("error out"=w190:T18, "array of 4 x 16 bit unsigned"=w188:u16[], "FrontPanel port"=w192:refnum<visa-resource-name>)  [unwired: 3 in]
            n111 = call "BP Query Delay.vi"("error in"=w190, "FrontPanel port"=w192) -> ("error out"=w189:T18, "array of 2 x 32 bit unsigned"=w187:u32[], "FrontPanel port"=w191:refnum<visa-resource-name>)  [unwired: 3 in]
            n112 = Array To Cluster(array=w188) -> (cluster=w193:T24)
            n113 = property on="P6&7 limits" class="Clust (strict)"("Value"=w193) -> ()  [unwired: 2 in, 2 out]
            n114 = Build Array (concatenate)(w188, w187) -> (w186:u32[])
            n115 = call "BP query P5.vi"("FrontPanel port"=w191) -> ("error out"=w196:T18, "array of 2 x 16 bit unsigned"=w201:u16[], "FrontPanel port"=w203:refnum<visa-resource-name>)  [unwired: 4 in]
            n116 = Greater Or Equal?(x=w207, y=4.0 ("x")) -> (x >= y?=w206:bool)
            n117 = Array To Cluster(array=w186) -> (cluster=w185:T25)
            n118 = Array To Cluster(array=w201) -> (cluster=w194:T26)
            n119 = Boolean To (0,1)(Boolean=w206) -> (0, 1=w205:i16)
            n120 = call "Disable on error.vi"("error out"=w196) -> ("Numeric"=w197:i16)
            n121 = call "BP query NCP5.vi"("FrontPanel port"=w203) -> ("error out"=w199:T18, "array of 3 x 16 bit unsigned"=w200:u16[], "FrontPanel port"=w202:refnum<visa-resource-name>)  [unwired: 4 in]
            n122 = property on="P6&7 Settings" class="Clust (strict)"("Value"=w185) -> ()  [unwired: 2 in, 2 out]
            n123 = property on="P5 Settings" class="Clust (strict)"("Value"=w194, "Disabled"=w197) -> ()  [unwired: 2 in, 2 out]
            n124 = property on="Tab Control 4" class="TabCtl (strict)"("Value"=w205) -> ()  [unwired: 2 in, 2 out]
            n125 = Array To Cluster(array=w200) -> (cluster=w195:T27)
            n126 = call "Disable on error.vi"("error out"=w199) -> ("Numeric"=w198:i16)
            n127 = property on="NCP5 Settings" class="Clust (strict)"("Value"=w195, "Disabled"=w198) -> ()  [unwired: 2 in, 2 out]
            n128 = property on="FP error" class="Clust (strict)"("Value"=w189) -> ()  [unwired: 2 in, 2 out]
            n129 = property on="P5 limits" class="Clust (strict)"("Value"=w194) -> ()  [unwired: 2 in, 2 out]
            n130 = property on="NCP5 limits" class="Clust (strict)"("Value"=w195) -> ()  [unwired: 2 in, 2 out]
          }
          frame #2 {
            n131 = property on="S2 Enabled?" class="Bool (strict)"() -> ("Value"=w218:bool)  [unwired: 2 in, 2 out]
            n132 = property on="S1 Enabled?" class="Bool (strict)"() -> ("Value"=w219:bool)  [unwired: 2 in, 2 out]
            n133 = case shown="False" w219 {
              tunnel: w222 -> [w226 w228]
              tunnel: [w226 w227] -> w217
              frame False {
              }
              frame True {
                n134 = call "PV Initialize.vi"("VISA session in"=w228) -> ("VISA session out"=w227:refnum<visa-resource-name>)  [unwired: 9 in, 1 out]
              }
            }
            n135 = case shown="False" w218 {
              tunnel: w221 -> [w223 w225]
              tunnel: [w223 w224] -> w220
              frame False {
              }
              frame True {
                n136 = call "PV Initialize.vi"("VISA session in"=w225) -> ("VISA session out"=w224:refnum<visa-resource-name>)  [unwired: 9 in, 1 out]
              }
            }
          }
          frame #3 {
            n137 = Tick Count (ms)() -> (millisecond timer value=w230:u32)
            n138 = Add(x=w230, y=u32 5000 ("Timer 1")) -> (x+y=w231:u32)
            n139 = local write "Timer 1"(w231) -> ()
            n140 = local write "Timer 2"(w231) -> ()
          }
          frame #4 {
            w232 = u8 0 ("Disabled")
            w234 = u8 0 ("Disabled")
            n141 = property on="Configuration" class="Clust (strict)"("Disabled"=u8 2) -> ()  [unwired: 2 in, 2 out]
            n142 = property on="Buttons" class="Clust"("Disabled"=w234) -> ()  [unwired: 2 in, 2 out]
            n143 = property on="Buttons 2" class="Clust"("Disabled"=w234) -> ()  [unwired: 2 in, 2 out]
            n144 = property on="Main Panel" class="TabCtl (strict)"("Disabled"=w232) -> ()  [unwired: 2 in, 2 out]
            n145 = property on="Error Panel" class="TabCtl (strict)"("Disabled"=w232) -> ()  [unwired: 2 in, 2 out]
            n146 = property on="Pressures Panel" class="TabCtl (strict)"("Disabled"=w232) -> ()  [unwired: 2 in, 2 out]
          }
          frame #5 {
            n147 = Set Occurrence(w235) -> ()
          }
        }
      }
      event "stop": Value Change {
        n148 = event-data() -> ()  [unwired: 1 in, 6 out]
        n149 = flat-sequence {
          tunnel: w236 -> [w242]
          tunnel: w240 -> [w245]
          tunnel: w239 -> [w243]
          tunnel: w238 -> [w244]
          tunnel: w237 -> [w246]
          frame #0 {
            n150 = Wait on Occurrence(2:w242) -> ()  [unwired: 2 in, 1 out]
          }
          frame #1 {
            n151 = VISA Close(VISA resource name=w245) -> ()  [unwired: 1 in, 1 out]
            n152 = VISA Close(VISA resource name=w243) -> ()  [unwired: 1 in, 1 out]
            n153 = VISA Close(VISA resource name=w244) -> ()  [unwired: 1 in, 1 out]
            n154 = VISA Close(VISA resource name=w246) -> ()  [unwired: 1 in, 1 out]
          }
          frame #2 {
            (unwired) T22."HKEY_CURRENT_USER" ("root key (HKEY_LOCAL_MACHINE) 2")
            n155 = control-ref of="Configuration"() -> (w251:refnum<vi>)
            n156 = control-ref of="ADC Scaling"() -> (w247:refnum<vi>)
            n157 = Build Array(w251, w247) -> (w253:refnum<vi>[])
            n158 = property on="Start" class="Bool"("Visible"=TRUE) -> ()  [unwired: 2 in, 2 out]
            n159 = call "Current VIs Parent Directory__ogtk.vi"("Relative path (.)"=path "config.ini") -> ("Parent Directory (+ Relative)"=w249:path)  [unwired: 4 in]
            n160 = call "Save Load Settings to File by Ref with path.vi"("Array of Cluster References"=w253, "subkey"="SOFTWARE\\Leiden Cryogenics\\FP" ("subkey 2"), "Action"=enum8{"Load", "Save"}."Save", "configuration file path"=w249) -> ()  [unwired: 5 in, 1 out]
          }
          frame #3 {
            n161 = property on="stop" class="Bool (strict)"("Value"=FALSE ("stop")) -> ()  [unwired: 2 in, 2 out]
          }
          frame #4 {
            n162 = Stop(stop? (T)=TRUE) -> ()
          }
        }
      }
      event "PT start": Value Change {
        w262 = u16 54529 items=["Compressor START"=54529, "Compressor STOP"=50584, "Error Code"=26020, "Reset Max/Min"=54235] ("Command")
        n163 = event-data() -> ()  [unwired: 1 in, 6 out]
        n164 = call "PT Send Command.vi"("Command"=w262, "Com Port #"=w259) -> ()  [unwired: 1 in, 2 out]
      }
      event "Buttons": Value Change {
        n165 = event-data() -> ("NewVal"=w272:T14)  [unwired: 1 in, 5 out]
        n166 = Cluster To Array(cluster=w272) -> (array=w271:bool[])
        n167 = while {
          tunnel: w271 -> [w274] mode=indexing
          tunnel: [w273] -> w270
          i -> [w273]
          stop <- w274 stop-if-true
        }
        n168 = Increment(x=w270) -> (x+1=w269:i32)
        n169 = call "BP togglekey.vi"("keynumber"=w269, "FrontPanel port"=w268) -> ("FrontPanel port"=w267:refnum<visa-resource-name>)  [unwired: 2 in, 1 out]
      }
      event "Buttons 2": Value Change {
        n170 = event-data() -> ("NewVal"=w284:T14)  [unwired: 1 in, 5 out]
        n171 = Cluster To Array(cluster=w284) -> (array=w283:bool[])
        n172 = while {
          tunnel: w283 -> [w286] mode=indexing
          tunnel: [w285] -> w282
          i -> [w285]
          stop <- w286 stop-if-true
        }
        n173 = Increment(x=w282) -> (x+1=w281:i32)
        n174 = call "BP togglekey.vi"("keynumber"=w281, "FrontPanel port"=w280) -> ("FrontPanel port"=w279:refnum<visa-resource-name>)  [unwired: 2 in, 1 out]
      }
      event "PT stop": Value Change {
        w292 = u16 50584 items=["Compressor START"=54529, "Compressor STOP"=50584, "Error Code"=26020, "Reset Max/Min"=54235] ("Command")
        n175 = event-data() -> ()  [unwired: 1 in, 1 out]
        n176 = call "PT Send Command.vi"("Command"=w292, "Com Port #"=w289) -> ()  [unwired: 1 in, 2 out]
      }
      event "PT Error Code": Value Change {
        n177 = event-data() -> ("OldVal"=w300:i32, "NewVal"=w296:i32)  [unwired: 1 in]
        n178 = Not Equal?(x=w300, y=w296) -> (x != y?=w299:bool)
        n179 = global read "ErrCodeStatusLkup.vi" "Error code/name/description Firmware V1.5"() -> (w297:string)
        n180 = case shown="Default" w296 {
          tunnel: w298 -> [_ w311]
          frame 0, 14..23 {
            # "No Error or Warning"
            "Attempts Counter" <- u16 0 ("Attempts Counter")
          }
          frame Default {
            # "Error"
            n181 = local read "Attempts Counter"() -> (w317:u16)
            n182 = Less?(x=w317, y="Attempts") -> (x < y?=w314:bool)
            n183 = And(x=w314, y="Restart PT on Error?") -> (x .and. y?=w313:bool)
            n184 = case shown="True" w313 {
              tunnel: "Time delay" -> [_ w319]
              tunnel: w311 -> [_ w318]
              frame False {
              }
              frame True {
                n185 = flat-sequence {
                  tunnel: w318 -> [w320]
                  tunnel: w319 -> [w324]
                  frame #0 {
                    n186 = call "PT start.vi"("Com Port #"=w320) -> ()  [unwired: 1 in, 2 out]
                  }
                  frame #1 {
                    n187 = local read "Attempts Counter"() -> (w322:u16)
                    n188 = Increment(x=w322) -> (x+1=w321:u16)
                    n189 = local write "Attempts Counter"(w321) -> ()
                  }
                  frame #2 {
                    n190 = Multiply(x=w324, y=u16 1000) -> (x*y=w325:u16)
                    n191 = Wait (ms)(milliseconds to wait=w325) -> ()  [unwired: 1 out]
                  }
                }
              }
            }
          }
        }
        n192 = Pick Line(multi-line string=w297, line index=w296) -> (output string=w295:string)  [unwired: 1 in]
        "PT Status" <- w295
        n193 = case shown="True" w299 {
          tunnel: w296 -> [_ w306]
          tunnel: w295 -> [_ w303]
          frame False {
          }
          frame True {
            n194 = Format Date/Time String() -> (date/time string=w304:string)  [unwired: 3 in]
            n195 = Number To Decimal String(number=w306) -> (decimal integer string=w305:string)  [unwired: 1 in]
            n196 = Build Array(w304, w305, w303) -> (w307:string[])
            n197 = feedback #5() -> (w308:string[][])  [unwired: 1 in]
            "Error Log" <- w308
            n198 = Build Array (concatenate)(w308, w307) -> (w309:string[][])
            n199 = feedback-in #5(w309) -> ()
          }
        }
      }
      event "Reset MIN/MAX": Value Change {
        w331 = u16 54235 items=["Compressor START"=54529, "Compressor STOP"=50584, "Error Code"=26020, "Reset Max/Min"=54235] ("Command")
        n200 = event-data() -> ()  [unwired: 1 in, 1 out]
        n201 = call "PT Send Command.vi"("Command"=w331, "Com Port #"=w328) -> ()  [unwired: 1 in, 2 out]
      }
      event "SET VALUES": Value Change {
        n202 = event-data() -> ("OldVal"=w356:bool, "NewVal"=w357:bool)  [unwired: 1 in, 4 out]
        n203 = property on="SET VALUES" class="Bool (strict)"("Value"=w356) -> ()  [unwired: 2 in, 2 out]
        n204 = call "BP Set Config.vi"("GHS Settings"="P6&7 Settings", "Set"=w357, "FrontPanel port"=w355) -> ("error out"=w337:T18, "FrontPanel port"=w349:refnum<visa-resource-name>)  [unwired: 1 in]
        n205 = call "BP Set P5.vi"("P5 Settings"="P5 Settings", "error in"=w337, "FrontPanel port in"=w349) -> ("error out"=w336:errorcluster, "FrontPanel port out"=w348:refnum<visa-resource-name>)  [unwired: 1 in]
        n206 = call "BP Set NCP5.vi"("NCP5 Settings"="NCP5 Settings", "error in"=w336, "FrontPanel port in"=w348) -> ("error out"=w335:errorcluster, "FrontPanel port out"=w339:refnum<visa-resource-name>)  [unwired: 1 in]
        n207 = call "BP query settings.vi"("error in"=w335, "FrontPanel port"=w339) -> ("error out"=w332:T18, "array of 4 x 16 bit unsigned"=w344:u16[], "FrontPanel port"=w333:refnum<visa-resource-name>)  [unwired: 3 in]
        n208 = call "BP query P5.vi"("error in"=w332, "FrontPanel port"=w333) -> ("error out"=w334:T18, "array of 2 x 16 bit unsigned"=w345:u16[], "FrontPanel port"=w342:refnum<visa-resource-name>)  [unwired: 3 in]
        n209 = call "BP query NCP5.vi"("error in"=w334, "FrontPanel port"=w342) -> ("array of 3 x 16 bit unsigned"=w346:u16[], "FrontPanel port"=w338:refnum<visa-resource-name>)  [unwired: 3 in, 1 out]
        n210 = Array To Cluster(array=w344) -> (cluster=→"P6&7 limits":T24)
        n211 = Array To Cluster(array=w345) -> (cluster=→"P5 limits":T26)
        n212 = Array To Cluster(array=w346) -> (cluster=→"NCP5 limits":T27)
      }
      event "Data Logging \nOptions.Plot data": Value Change {
        n213 = event-data() -> ("NewVal"=w364:bool)  [unwired: 1 in, 5 out]
        n214 = property on="Main Panel" class="TabCtl (strict)"() -> ("Pages"=w367:refnum<vi>[])  [unwired: 2 in, 2 out]
        n215 = Index Array(array=w367, index=2) -> (element=w365:refnum<vi>)
        n216 = property class="Page"(reference=w365, "PageVis"=w364) -> ()  [unwired: 1 in, 2 out]
      }
      event "Autoconf": Value Change {
        n217 = event-data() -> ()  [unwired: 1 in, 6 out]
      }
      event "Configuration": Value Change {
        n218 = event-data() -> ("NewVal"=w379:T12)  [unwired: 1 in, 5 out]
        n219 = Unbundle By Name(w379) -> ("Type"=w378:enum32{"CF", "Wet"})
        n220 = VISA Close(VISA resource name=w387) -> ()  [unwired: 1 in, 1 out]
        n221 = VISA Close(VISA resource name=w388) -> ()  [unwired: 1 in, 1 out]
        n222 = VISA Close(VISA resource name=w376) -> ()  [unwired: 1 in, 1 out]
        n223 = VISA Close(VISA resource name=w374) -> ()  [unwired: 1 in, 1 out]
        n224 = case shown="\"CF\", Default" w378 {
          tunnel: ["COMPRESSOR" ("Label.Text") "AUX 2" ("Label.Text")] -> w386
          tunnel: [TRUE ("Visible") FALSE ("Visible")] -> w382
          tunnel: ["From\nProbe" ("Text.Text") "From\nDewar" ("Text.Text")] -> w381
          tunnel: ["From\nOVC" ("Text.Text") "From\n1K pot" ("Text.Text")] -> w380
          frame "CF", Default {
          }
          frame "Wet" {
          }
        }
        n225 = Unbundle By Name("Configuration") -> ("PT port"=w391:refnum<visa-resource-name>, "FP port"=w392:refnum<visa-resource-name>, "MG port"=w377:refnum<visa-resource-name>, "S1 port"=w375:refnum<visa-resource-name>, "S2 port"=w373:refnum<visa-resource-name>)
        n226 = property on="Main Panel" class="TabCtl (strict)"() -> ("Pages"=w385:refnum<vi>[])  [unwired: 2 in, 2 out]
        n227 = Index Array(array=w385, index=1) -> (element=w383:refnum<vi>)
        n228 = property on="COMPR/AUX 2" class="Bool (strict)"("Caption.Text"=w386) -> ()  [unwired: 2 in, 2 out]
        n229 = property on="String 3" class="Str"("Text.Text"=w381) -> ()  [unwired: 2 in, 2 out]
        n230 = property on="String" class="Str"("Text.Text"=w380) -> ()  [unwired: 2 in, 2 out]
        n231 = call "VISA to RS232 Port Nr.vi"("VISA Resource Name"=w391) -> ("Port Number"=w390:u8)  [unwired: 1 in]
        n232 = property on="BYPASS" class="Bool (strict)"("Visible"=w382) -> ()  [unwired: 2 in, 2 out]
        n233 = property on="PT STATUS" class="Bool (strict)"("Visible"=w382) -> ()  [unwired: 2 in, 2 out]
        n234 = property class="Page"(reference=w383, "PageVis"=w382) -> ()  [unwired: 1 in, 2 out]
        n235 = Increment(x=w390) -> (x+1=w389:u8)
      }
      event "Configuration.Type": Value Change {
        n236 = event-data() -> ()  [unwired: 1 in, 6 out]
      }
      event "FP Status bits": Value Change {
        n237 = event-data() -> ("OldVal"=w414:u32[], "NewVal"=w413:u32[])  [unwired: 1 in, 4 out]
        n238 = Not Equal?(x=w414, y=w413) -> (x != y?=w412:bool)
        n239 = case shown="True" w412 {
          frame False {
          }
          frame True {
            w415 = u32 0 ("timer")
            n240 = local write "Timer 1"(w415) -> ()
            n241 = local write "Timer 2"(w415) -> ()
          }
        }
      }
      event "Front Panel", "MaxiGauge": Shortcut Menu Activation? {
        w423 = string[] ["Zoom In to Last Data", "Autoscale XY"] ("item names")
        n242 = event-data() -> ("MenuRef"=w421:refnum<k9>)  [unwired: 1 in, 6 out]
        n243 = Insert Menu Items(4:10, 7:w423, 8:w423, 9:w421) -> ()  [unwired: 2 in, 3 out]
        n244 = event-data() -> ()  [unwired: 2 in, 1 out]
      }
      event "Front Panel", "MaxiGauge": Shortcut Menu Selection (User) {
        n245 = event-data() -> ("CtlRef"=w431:refnum<vi>, "ItemTag"=w430:string)  [unwired: 1 in, 6 out]
        n246 = Type Cast(type=refnum<vi> refnum ("R-Plot 0"), x=w431) -> (*(type *) &x=w429:refnum<vi>)
        n247 = case shown="\"Zoom In to Last Data\"" w430 {
          tunnel: w429 -> [_ w433 w435]
          frame Default {
          }
          frame "Autoscale XY" {
            w434 = u8 2 ("X Scale.Scale Fit")
            n248 = property class="XYGraph (strict)"(reference=w433, "XScale.ScaleFit"=w434, "YScale.ScaleFit"=w434) -> ()  [unwired: 1 in, 2 out]
          }
          frame "Zoom In to Last Data" {
            w440 = u8 0 ("Y Scale.Scale Fit")
            n249 = property class="XYGraph (strict)"(reference=w435) -> (reference out=w439:refnum<vi>, "Value"=w437:cluster{dbl[], dbl[]})  [unwired: 1 in, 1 out]
            n250 = Unbundle(w437) -> (w461:dbl[], w438:dbl[])
            n251 = Multiply(x=15.0, y=60.0) -> (x*y=w444:dbl)
            n252 = Reverse 1D Array(array=w461) -> (reversed array=w456:dbl[])
            n253 = Reverse 1D Array(array=w438) -> (reversed array=w448:dbl[])
            n254 = Index Array(array=w456) -> (element=w442:dbl)  [unwired: 1 in]
            n255 = Multiply(x=0.5, y=w444) -> (x*y=w443:dbl)
            n256 = Add(x=w443, y=w442) -> (x+y=w445:dbl)
            n257 = Subtract(x=w442, y=w444) -> (x-y=w447:dbl)
            n258 = call "Improved Threshold Detector.71.vi"("Threshold"=w447, "Array"=w461) -> ("Positive transition indices"=w460:i32[])  [unwired: 8 in, 1 out]
            n259 = Index Array(array=w460) -> (element=w436:i32)  [unwired: 1 in]
            n260 = Array Size(array=w461) -> (size(s)=w458:i32)
            n261 = Index Array(array=w461, index=w436) -> (element=w462:dbl)
            n262 = Subtract(x=w458, y=w436) -> (x-y=w459:i32)
            n263 = Array Subset(array=w448, length=w459) -> (w449:dbl[])  [unwired: 1 in]
            n264 = Array Max & Min(array=w449) -> (max value=w452:dbl, min value=w453:dbl)  [unwired: 2 out]
            n265 = Subtract(x=w452, y=w453) -> (x-y=w450:dbl)
            n266 = Divide(x=w450, y=2.0) -> (x/y=w454:dbl)
            n267 = Add(x=w452, y=w454) -> (x+y=w457:dbl)
            n268 = Subtract(x=w453, y=w454) -> (x-y=w455:dbl)
            n269 = property class="XYGraph (strict)"(reference=w439, "XScale.ScaleFit"=w440, "YScale.ScaleFit"=w440, "XScale.Maximum"=w445, "XScale.Minimum"=w462, "YScale.Maximum"=w457, "YScale.Minimum"=w455) -> ()  [unwired: 1 in, 2 out]
          }
        }
      }
      event "Reset Error": Value Change {
        n270 = event-data() -> ()  [unwired: 1 in, 6 out]
        n271 = property on="Device address S1" class="DigNum (strict)"() -> ("Value"=w464:u8)  [unwired: 2 in, 2 out]
        n272 = call "PV Error Reset.vi"("Adress of unit"=w464, "VISA session"=w469) -> ()  [unwired: 8 in, 2 out]
      }
      event "Reset Error 2": Value Change {
        n273 = event-data() -> ()  [unwired: 1 in, 6 out]
        n274 = property on="Device address S2" class="DigNum (strict)"() -> ("Value"=w470:u8)  [unwired: 2 in, 2 out]
        n275 = call "PV Error Reset.vi"("Adress of unit"=w470, "VISA session"=w475) -> ()  [unwired: 8 in, 2 out]
      }
      event "Configuration.S1 Enabled?": Value Change {
        n276 = event-data() -> ("NewVal"=w485:bool)  [unwired: 1 in, 5 out]
        n277 = Not(x=w485) -> (.not. x?=w484:bool)
        n278 = Boolean To (0,1)(Boolean=w484) -> (0, 1=w483:i16)
        n279 = Multiply(x=i16 2, y=w483) -> (x*y=w481:i16)
        n280 = property on="S1" class="TabCtl (strict)"("Disabled"=w481) -> ()  [unwired: 2 in, 2 out]
      }
      event "Configuration.S2 Enabled?": Value Change {
        n281 = event-data() -> ("NewVal"=w492:bool)  [unwired: 1 in, 5 out]
        n282 = Not(x=w492) -> (.not. x?=w495:bool)
        n283 = Boolean To (0,1)(Boolean=w495) -> (0, 1=w494:i16)
        n284 = Multiply(x=i16 2, y=w494) -> (x*y=w491:i16)
        n285 = property on="S2" class="TabCtl (strict)"("Disabled"=w491) -> ()  [unwired: 2 in, 2 out]
      }
    }
  }
  n286 = flat-sequence {
    tunnel: w4 -> [w496]
    tunnel: w1 -> [w633]
    frame #0 {
      n287 = Wait on Occurrence(2:w496) -> ()  [unwired: 2 in, 1 out]
    }
    frame #1 {
      n288 = property on="PT Enabled?" class="Bool (strict)"() -> ("Value"=w500:bool)  [unwired: 2 in, 2 out]
      n289 = while {
        stop <- "stop" stop-if-true
        n290 = property on="FP error" class="Clust (strict)" props=["Value"]() -> (error out=w524:errorcluster)  [unwired: 2 in, 2 out]
        n291 = property on="FP port" class="VISAName"() -> ("Value"=w525:refnum<visa-resource-name>)  [unwired: 2 in, 2 out]
        n292 = stacked-sequence {
          seq-local: [w549 _ _] -> [_ w560 _]
          seq-local: [w548 _ _] -> [_ w559 _]
          seq-local: [_ w552 _] -> [_ _ w582]
          seq-local: [_ w553 _] -> [_ _ w581]
          tunnel: [_ _ w580] -> w528
          tunnel: w524 -> [w546 _ _]
          tunnel: [_ _ w579] -> w527
          tunnel: w525 -> [w547 _ _]
          frame #0 {
            # "PT on"
            n293 = call "BP Query KeyStatus.vi"("error in"=w546, "FrontPanel port"=w547) -> ("error out"=w549:T18, "boolean array of keyvalues"=w545:bool[], "FrontPanel port"=w548:refnum<visa-resource-name>)  [unwired: 3 in]
            n294 = Build Array (concatenate)(w545, FALSE) -> (w531:bool[])
            n295 = Array To Cluster(array=w531) -> (cluster=→"LEDs" →"LEDs 2":T28)
            n296 = Array Subset(array=w531, index=0, length=32) -> (w540:bool[])
            n297 = Array Subset(array=w531, index=32, length=32) -> (w537:bool[])
            n298 = Array Subset(array=w531, index=64, length=32) -> (w543:bool[])
            n299 = Boolean Array To Number(Boolean array=w540) -> (number=w533:u32)
            n300 = Boolean Array To Number(Boolean array=w537) -> (number=w534:u32)
            n301 = Boolean Array To Number(Boolean array=w543) -> (number=w532:u32)
            n302 = Build Array(w533, w534, w532) -> (w530:u32[])
            n303 = property on="FP Status bits" class="Arr (strict)"("Val(Sgnl)"=w530) -> ()  [unwired: 2 in, 2 out]
          }
          frame #1 {
            # "input range Pstill for DR blindpanel: 16 bit unsigned, FullScale is 10mBar"
            n304 = local read "Pstill (P8)"() -> (w558:dbl)
            n305 = call "BP Query Status.vi"("error in"=w560, "FrontPanel port"=w559) -> ("error out"=w550:T18, "status word (32 bit unsigned)"=w569:u32, "FrontPanel port"=w551:refnum<visa-resource-name>)  [unwired: 3 in]
            n306 = property on="Read P8" class="Bool (strict)"() -> ("Value"=w556:bool)  [unwired: 2 in, 2 out]
            n307 = Divide(x=65535, y=10) -> (x/y=w561:dbl)
            n308 = Select(t=w558, s=w556, f=1000.0) -> (s? t:f=w555:dbl)
            n309 = Multiply(x=w561, y=w555) -> (x*y=w563:dbl)
            n310 = And(x=w569, y=u16 7) -> (x .and. y?=→"Mode":u32)
            n311 = And(x=u32 65536, y=w569) -> (x .and. y?=w564:u32)
            n312 = To Unsigned Word Integer(number=w563) -> (unsigned 16bit integer=w562:u16)
            n313 = Not Equal To 0?(x=w564) -> (x != 0?=w554:bool)
            n314 = call "BP Send Values.vi"("error in"=w550, "value to send"=w562, "FrontPanel port"=w551) -> ("error out"=w552:T18, "FrontPanel port"=w553:refnum<visa-resource-name>)  [unwired: 3 in]
            n315 = property on="P5 Alarm" class="Bool (strict)"("Blinking"=w554, "Value"=w554) -> ()  [unwired: 2 in, 2 out]
          }
          frame #2 {
            # "adc channels (P1..P7,Flow,PC,..)"
            n316 = Unbundle By Name("ADC Scaling") -> ("Front panel ADC scaling factors"=w576:T29)
            n317 = Cluster To Array(cluster=w576) -> (array=w575:dbl[])
            n318 = call "BP Query Adc.vi"("error in"=w582, "FrontPanel port"=w581) -> ("error out"=w579:T18, "array of 8 x 16 bit unsigned"=w574:i32[], "FrontPanel port"=w580:refnum<visa-resource-name>)  [unwired: 3 in]
            n319 = property on="Averages" class="DigNum (strict)"() -> ("Value"=w573:i32)  [unwired: 2 in, 2 out]
            n320 = call "BP Scale Adc-NEW PANEL.vi"("input array 8 x 16bit uint"=w574, "input array scaling factors, 7 x 16 bit uint"=w575) -> ("output array 8 x single prec. incl flow"=w578:sgl[])  [unwired: 2 in, 1 out]
            n321 = call "Running average.vi"("Window Size"=w573, "New values"=w578, "Filter Zeroes? (T)"=FALSE) -> ("Filterred"=→"FP Data":dbl[])  [unwired: 1 in]
          }
        }
        "FP error" <- w527
        n322 = Wait (ms)(milliseconds to wait=u32 250) -> ()  [unwired: 1 out]
        n323 = call "MGI Milliseconds Since Last Call.vi"() -> ("ms"=→"millisecond timer value":u32)  [unwired: 6 in, 1 out]
        n324 = property on="FP port" class="VISAName"("Value"=w528) -> ()  [unwired: 2 in, 2 out]
      }
      n325 = property on="PT Slave \nAddress" class="DigNum (strict)"() -> ("Value"=w501:u8)  [unwired: 2 in, 2 out]
      n326 = property on="PT port" class="VISAName"() -> ("Value"=w504:refnum<visa-resource-name>)  [unwired: 2 in, 2 out]
      n327 = call "VISA to RS232 Port Nr.vi"("VISA Resource Name"=w504) -> ("Port Number"=w503:u8)  [unwired: 1 in]
      n328 = Increment(x=w503) -> (x+1=w502:u8)
      n329 = while {
        tunnel: w502 -> [w606]
        tunnel: w501 -> [w605]
        tunnel: w500 -> [w603]
        stop <- w601 stop-if-true
        n330 = case shown="False" w603 {
          tunnel: [dbl[] [0.0, 0.0, 0.0, 0.0, 0.0, 0.0, 0.0, 0.0] w615] -> w608
          tunnel: w606 -> [_ w614]
          tunnel: errorcluster {"status"=FALSE, "code"=0, "source"=""} ("error in (no error)") -> [_ w613]
          tunnel: w605 -> [_ w611]
          frame False {
          }
          frame True {
            n331 = call "PT Read Status.vi"("error in (no error)"=w613, "Slave Address"=w611, "Com Port #"=w614) -> ("error out"=→"PT error":errorcluster, "Response"=w616:T30)
            n332 = call "PT Parse Response.vi"("Response"=w616) -> ("Oil temp"=w621:T31, "Pressure"=w626:T32, "He temp"=w620:T33, "Out water temp"=w619:T34, "Numeric"=w630:i32, "In water temp"=w618:T35, "Current"=w627:i32, "PT Error"=w617:i32)
            "Oil Temp" <- w621
            "Motor Current" <- w627
            "PT Control" <- w630
            "Out Water Temp" <- w619
            "He Pressure" <- w626
            "In Water Temp" <- w618
            "He Temp" <- w620
            n333 = property on="PT Error" class="DigNum (strict)"("Val(Sgnl)"=w617) -> ()  [unwired: 2 in, 2 out]
            n334 = Not Equal To 0?(x=w630) -> (x != 0?=w631:bool)
            n335 = Unbundle By Name(w618) -> ("Values[0]"=w625:dbl)
            n336 = Unbundle By Name(w626) -> ("[0]"=w628:dbl, "[1]"=w629:dbl)
            n337 = Unbundle By Name(w619) -> ("[1]"=w624:dbl)
            n338 = Unbundle By Name(w620) -> ("[2]"=w623:dbl)
            n339 = Unbundle By Name(w621) -> ("[3]"=w622:dbl)
            n340 = Boolean To (0,1)(Boolean=w631) -> (0, 1=w632:i16)
            n341 = Build Array(w632, w625, w624, w623, w622, w628, w629, w627) -> (w615:dbl[])
          }
        }
        n342 = local read "stop"() -> (w601:bool)
        n343 = property on="Averages" class="DigNum (strict)"() -> ("Value"=w604:i32)  [unwired: 2 in, 2 out]
        n344 = call "Running average.vi"("Window Size"=w604, "New values"=w608) -> ("Filterred"=→"PT Data":dbl[])  [unwired: 2 in]
        n345 = Wait (ms)(milliseconds to wait=u32 250) -> ()  [unwired: 1 out]
      }
      n346 = property on="S1?" class="Bool (strict)"() -> ("Value"=w499:bool)  [unwired: 2 in, 2 out]
      n347 = while {
        tunnel: w499 -> [w593]
        stop <- w592 stop-if-true
        n348 = case shown="False" w593 {
          frame False {
          }
          frame True {
            n349 = property on="S1 port" class="VISAName"() -> ("Value"=w600:refnum<visa-resource-name>)  [unwired: 2 in, 2 out]
            n350 = property on="Device address S1" class="DigNum (strict)"() -> ("Value"=w595:u8)  [unwired: 2 in, 2 out]
            n351 = call "HiPACE status.vi"("Port"=w600, "Device address"=w595) -> ("Turbo status"=→"Turbo status":T36, "Turbo IW"=→"Turbo IW":cluster{"I:":string, "P:":string}, "Turbo T"=→"Turbo T":T4, "Error code"=→"Error code":string)  [unwired: 9 in, 1 out]
          }
        }
        n352 = Wait (ms)(milliseconds to wait=u32 500) -> ()  [unwired: 1 out]
        n353 = local read "stop"() -> (w592:bool)
      }
      n354 = property on="MG Enabled?" class="Bool (strict)"() -> ("Value"=w497:bool)  [unwired: 2 in, 2 out]
      n355 = while {
        shift-right: [w509] -> _
        shift-left: _ -> [w514]
        tunnel: w497 -> [w507]
        stop <- w505 stop-if-true
        n356 = property on="MG port" class="VISAName"() -> ("Value"=w513:refnum<visa-resource-name>)  [unwired: 2 in, 2 out]
        n357 = call "MG collect pressureinfo.vi"("error in"=w514, "VI action"=w507, "MaxiGauge port"=w513) -> ("sensor values"=w510:dbl[], "error out"=w516:T37, "sensor status info"=w519:string[], "MaxiGauge port"=w521:refnum<visa-resource-name>)  [unwired: 2 out]
        n358 = Array To Cluster(array=w519) -> (cluster=→"Sensors Status":T38)
        n359 = property on="Averages" class="DigNum (strict)"() -> ("Value"=w508:i32)  [unwired: 2 in, 2 out]
        n360 = call "Running average.vi"("Window Size"=w508, "New values"=w510) -> ("Filterred"=w506:dbl[])  [unwired: 2 in]
        "MG Data" <- w506
        n361 = call "MG get errorstatus.vi"("error in"=w516, "VI action"=w507, "MaxiGauge port"=w521) -> ("error out"=w509:T37, "Sensor error status"=→"Sensor ERROR":string, "MaxiGauge error status"=→"MaxiGauge ERROR":string, "MaxiGauge port"=w512:refnum<visa-resource-name>)  [unwired: 1 in]
        "MG error" <- w509
        n362 = Array To Cluster(array=w506) -> (cluster=→"cluster":T39)
        n363 = local read "stop"() -> (w505:bool)
        n364 = property on="MG port" class="VISAName"("Value"=w512) -> ()  [unwired: 2 in, 2 out]
        n365 = Wait (ms)(milliseconds to wait=u32 500) -> ()  [unwired: 1 out]
      }
      n366 = property on="S2?" class="Bool (strict)"() -> ("Value"=w498:bool)  [unwired: 2 in, 2 out]
      n367 = while {
        tunnel: w498 -> [w584]
        stop <- w583 stop-if-true
        n368 = case shown="False" w584 {
          frame False {
          }
          frame True {
            n369 = property on="S2 port" class="VISAName"() -> ("Value"=w591:refnum<visa-resource-name>)  [unwired: 2 in, 2 out]
            n370 = property on="Device address S2" class="DigNum (strict)"() -> ("Value"=w586:u8)  [unwired: 2 in, 2 out]
            n371 = call "HiPACE status.vi"("Port"=w591, "Device address"=w586) -> ("Turbo status"=→"Turbo status 2":T36, "Turbo IW"=→"Turbo IW 2":cluster{"I:":string, "P:":string}, "Turbo T"=→"Turbo T 2":T4, "Error code"=→"Error code":string)  [unwired: 9 in, 1 out]
          }
        }
        n372 = Wait (ms)(milliseconds to wait=u32 500) -> ()  [unwired: 1 out]
        n373 = local read "stop"() -> (w583:bool)
      }
    }
    frame #2 {
      n374 = Set Occurrence(w633) -> ()
    }
  }
